vi "Open_test_database.vi"(8 "error in (no error)":errorcluster) -> (0 "error out":errorcluster, 3 "SQL conn Refnum out":refnum<k7>)   [LabVIEW 2013]
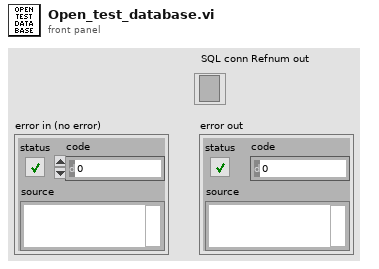
[diagram p1: front panel]
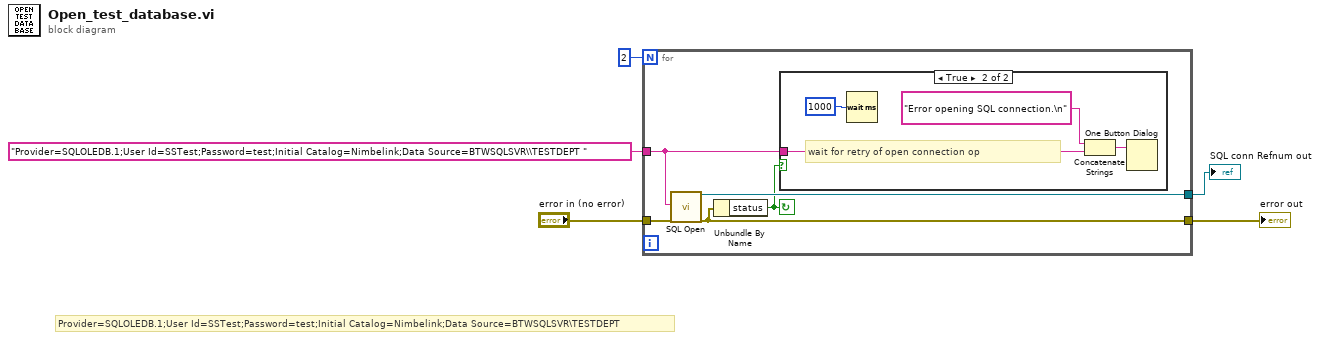
[diagram p0: block diagram]
diagram:
  # "Provider=SQLOLEDB.1;User Id=SSTest;Password=test;Initial Catalog=Nimbelink;Data Source=BTWSQLSVR\\TESTDEPT"
  n1 = for {
    N: 2 -> [_]
    tunnel: "error in (no error)" -> [w10]
    tunnel: [w8] -> w1
    tunnel: [w9] -> w2
    tunnel: "Provider=SQLOLEDB.1;User Id=SSTest;Password=test;Initial Catalog=Nimbelink;Data Source=BTWSQLSVR\\TESTDEPT " -> [w6]
    stop <- w7 continue-if-true
    n2 = call "SQL Open.vi"("ConnectionString In"=w6, "Error in (no error)"=w10) -> ("Connection Out"=w9:refnum<k7>, "Error out"=w8:errorcluster)  [unwired: 16 in]
    n3 = Unbundle By Name(w8) -> ("status"=w7:bool)
    n4 = case shown="True" w7 {
      tunnel: w6 -> [_ w11]
      frame False {
        # "open good"
      }
      frame True {
        # "wait for retry of open connection op"
        n5 = Wait (ms)(milliseconds to wait=u32 1000) -> ()  [unwired: 1 out]
        n6 = Concatenate Strings("Error opening SQL connection.\n" ("string"), w11) -> (w13:string)
        n7 = One Button Dialog(message=w13) -> ()  [unwired: 1 in, 1 out]
      }
    }
  }
  "SQL conn Refnum out" <- w2
  "error out" <- w1
